vi "GetStopEMG-Queuevi.vi"(8 "error in (no error)":errorcluster, 11 "EMGStop":refnum<queue>) -> (0 "error out":errorcluster, 3 "StopOut":bool)   [LabVIEW 2017]
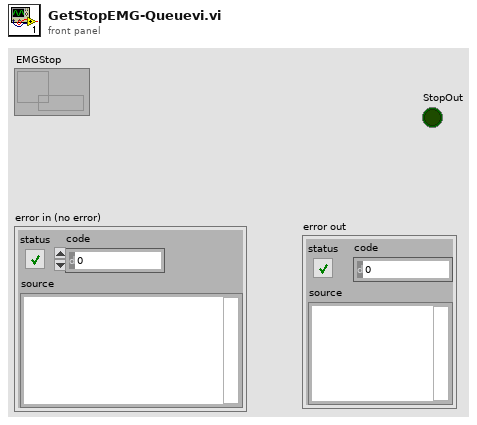
[diagram p1: front panel]
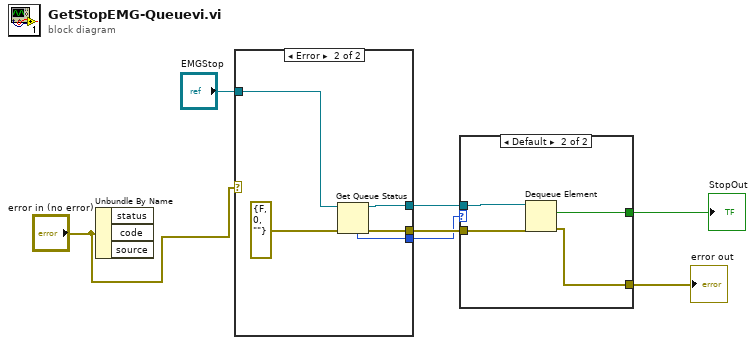
[diagram p0: block diagram]
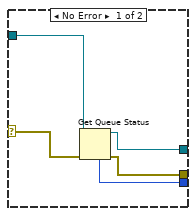
[diagram p2: hidden frame]
diagram:
  n1 = Unbundle By Name("error in (no error)") -> ()  [unwired: 3 out]
  n2 = case shown="Error" "error in (no error)" {
    selector: "error in (no error)" -> [w12 _]
    tunnel: "EMGStop" -> [w9 w17]
    tunnel: [w10 w16] -> w6
    tunnel: [w11 w15] -> w4
    tunnel: [w8 w14] -> w2
    frame No Error {
      n3 = Get Queue Status(queue=w9, error in (no error)=w12) -> (queue out=w10:refnum<queue>, error out=w11:errorcluster, # elements in queue=w8:i32)  [unwired: 1 in, 5 out]
    }
    frame Error {
      n4 = Get Queue Status(queue=w17, error in (no error)=errorcluster {"status"=FALSE, "code"=0, "source"=""}) -> (queue out=w16:refnum<queue>, error out=w15:errorcluster, # elements in queue=w14:i32)  [unwired: 1 in, 5 out]
    }
  }
  n5 = case shown="Default" w2 {
    tunnel: w6 -> [_ w22]
    tunnel: [_ w21] -> w5
    tunnel: w4 -> [w18 w20]
    tunnel: [w18 w19] -> w3
    frame 0 {
    }
    frame Default {
      n6 = Dequeue Element(queue=w22, error in (no error)=w20) -> (element=w21:bool, error out=w19:errorcluster)  [unwired: 1 in, 2 out]
    }
  }
  "StopOut" <- w5
  "error out" <- w3
